vi "replace by name.vi"(8 "error in (no error)":errorcluster, 10 "New object":refnum<class "system object.lvclass">, 11 "SysObj in":refnum<class "system object.lvclass">) -> (0 "error out":errorcluster, 1 "Replaced":bool, 3 "SysObj out":refnum<class "system object.lvclass">)   [LabVIEW 2020, in "system object.lvclass"]
uses:
  system object.lvclass
  system object.lvclass/system object.ctl
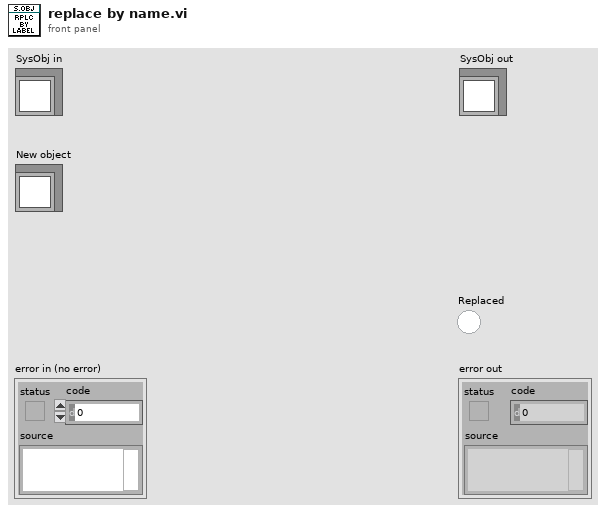
[diagram p1: front panel]
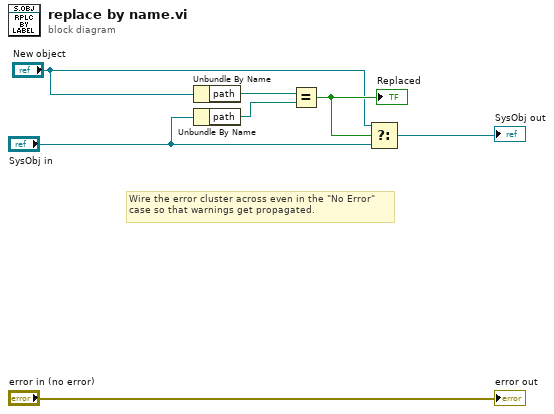
[diagram p0: block diagram]
diagram:
  # "Wire the error cluster across even in the \"No Error\"\ncase so that warnings get propagated."
  n1 = Unbundle By Name("New object") -> ("path"=w6:path)
  n2 = Unbundle By Name("SysObj in") -> ("path"=w5:path)
  n3 = Equal?(x=w6, y=w5) -> (x = y?=w4:bool)
  "Replaced" <- w4
  n4 = Select(t="New object", s=w4, f="SysObj in") -> (s? t:f=→"SysObj out":refnum<class "system object.lvclass">)
  "error out" <- "error in (no error)"
